vi "Connection Input Dialog.vi"(8 "Error in":errorcluster caption="Error in (no error)", 11 "Connection Info":cluster{"IP Address":string, "Port":u16}) -> (0 "Error out":errorcluster, 3 "Connection Info output":cluster{"IP Address":string, "Port":u16})   [LabVIEW 2020]
uses:
  1a42c072-7bdb-4d1e-a543-4b3cdf6af97b.vi
  b1d91e31-0c0c-4a7c-a377-974e3feb003e.vi
  1a42c072-7bdb-4d1e-a543-4b3cdf6af97b.vi/b09b9099-6be0-413b-8afc-4908471460c3.vi
  <userlib>/_NEVSTOP/Communicable State Machine(CSM)/addons/INI-Static-Variable-Support/_Support/FlagInstance-CSMINIVariable.vi
  b1d91e31-0c0c-4a7c-a377-974e3feb003e.vi/99de0c97-112a-4c86-9094-c187659127e1.vi
  <vilib>/Utility/error.llb/Clear Errors.vi
  <userlib>/_NEVSTOP/Communicable State Machine(CSM)/_Support/ChangeFlag/ChangeFlag-Read.vi
  <userlib>/_NEVSTOP/Communicable State Machine(CSM)/_Support/ChangeFlag/ChangeFlagDB.vi
  <vilib>/Utility/Data Type/Get Type Information.vi
  <userlib>/_NEVSTOP/Communicable State Machine(CSM)/addons/API-String-Arugments-Support/_Support/Data To SingleElementsArray_csm.vi
  <userlib>/_NEVSTOP/Communicable State Machine(CSM)/addons/INI-Static-Variable-Support/_Support/Parse Used Session and Name.vi
  <userlib>/_NEVSTOP/Communicable State Machine(CSM)/addons/API-String-Arugments-Support/_Support/Data To API String Arguments.vi
  <userlib>/_NEVSTOP/Communicable State Machine(CSM)/addons/INI-Static-Variable-Support/_Support/INI-FGV(lvlibp).vi
  <userlib>/_NEVSTOP/Communicable State Machine(CSM)/addons/INI-Static-Variable-Support/_Support/Populate String with INI Variable.vi
  <userlib>/_NEVSTOP/Communicable State Machine(CSM)/addons/API-String-Arugments-Support/_Support/Convert API String Arguments to Data(variant).vi
  <userlib>/_NEVSTOP/Communicable State Machine(CSM)/addons/API-String-Arugments-Support/_Support/SingleElementsArray To Data_csm.vi
panel:
  in  "Connect":bool
  in  "Port":u16=50007
  in  "IP Address":string="localhost"
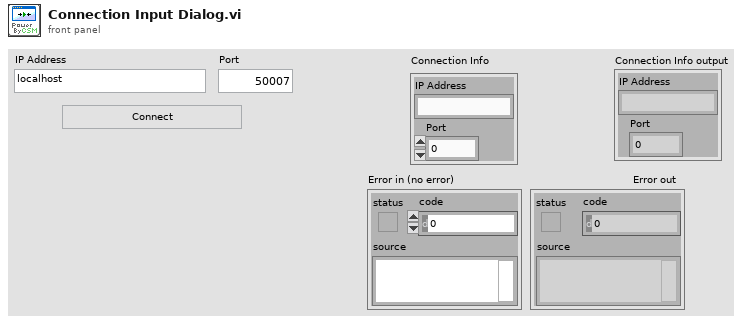
[diagram p1: front panel]
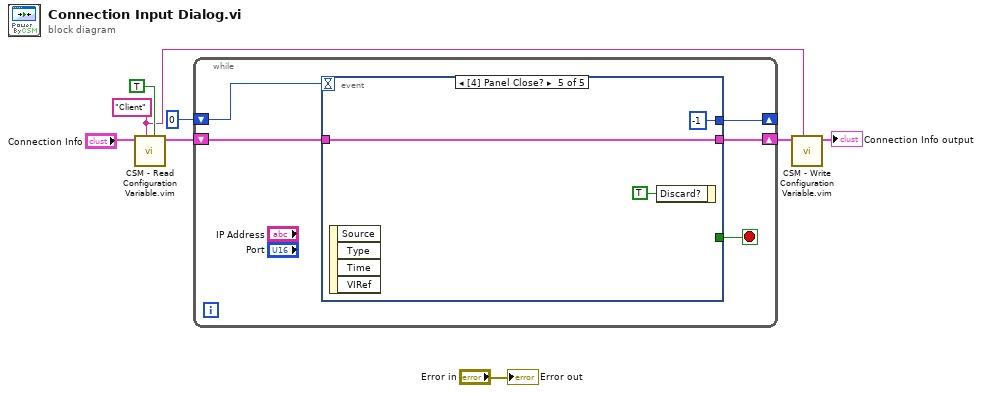
[diagram p0: block diagram]
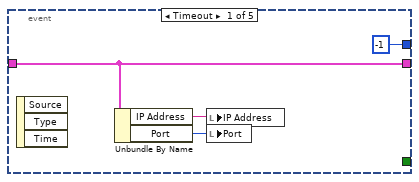
[diagram p2: hidden frame]
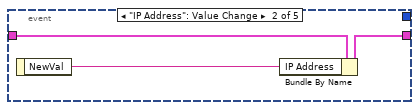
[diagram p3: hidden frame]
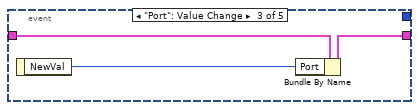
[diagram p4: hidden frame]
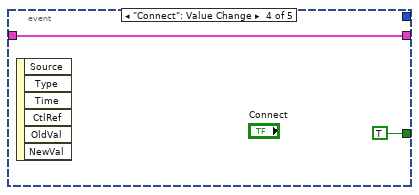
[diagram p5: hidden frame]
diagram:
  w1 = "Client" ("Section Name(\"\" as Default)")
  n1 = call "CSM - Read Configuration Variable.vim"("Write If not found?(F)"=TRUE, "Section Name(\"\" as Default)"=w1, "config prototype(Cluster Prefered)"="Connection Info") -> ("config out"=w8:cluster{"IP Address":string, "Port":u16})  [unwired: 5 in, 1 out]
  n2 = while {
    shift-right: [w10] -> _
    shift-left: 0 -> [w13]
    shift-right: [w11] -> w3
    shift-left: w8 -> [w12]
    stop <- w9 stop-if-true
    n3 = event shown="[4] Panel Close?" {
      selector: _ -> [_ _ _ _ _]
      dyn-events: _ -> [_ _ _ _ _]
      timeout: w13 -> [_ _ _ _ _]
      tunnel: w12 -> [w16 w20 w23 w25 w27]
      tunnel: [w16 w19 w22 w25 w27] -> w11
      tunnel: [-1 _ _ _ -1] -> w10
      tunnel: [_ _ _ TRUE _] -> w9
      event Timeout {
        n4 = event-data() -> ()  [unwired: 1 in, 3 out]
        n5 = Unbundle By Name(w16) -> ("IP Address"=w14:string, "Port"=w15:u16)
        n6 = local write "IP Address"(w14) -> ()
        n7 = local write "Port"(w15) -> ()
      }
      event "IP Address": Value Change {
        n8 = event-data() -> ("NewVal"=w18:string)  [unwired: 1 in]
        n9 = Bundle By Name(cluster=w20, "IP Address"=w18) -> (w19:cluster{"IP Address":string, "Port":u16})
      }
      event "Port": Value Change {
        n10 = event-data() -> ("NewVal"=w21:u16)  [unwired: 1 in]
        n11 = Bundle By Name(cluster=w23, "Port"=w21) -> (w22:cluster{"IP Address":string, "Port":u16})
      }
      event "Connect": Value Change {
        n12 = event-data() -> ()  [unwired: 1 in, 6 out]
      }
      event Panel Close? {
        n13 = event-data() -> ()  [unwired: 1 in, 4 out]
        n14 = event-data("Discard?"=TRUE) -> ()  [unwired: 1 in, 1 out]
      }
    }
  }
  n15 = call "CSM - Write Configuration Variable.vim"("Section Name(\"\" as Default)"=w1, "Variant"=w3) -> ("Variant (dup)"=→"Connection Info output":cluster{"IP Address":string, "Port":u16})  [unwired: 6 in, 1 out]
  "Error out" <- "Error in"
